vi "setMode.vi"(8 "error in (no error)":errorcluster, 10 "Mode":T1, 11 "Multimeter in":refnum<class "Multimeter.lvclass">) -> (0 "error out":errorcluster, 3 "Multimeter out":refnum<class "Multimeter.lvclass">)   [LabVIEW 2023, in "sweDmm.lvlib" / "Multimeter.lvclass"]
doc: "specify what the Dmm should measure."
uses:
  Multimeter.lvclass
  Data/DmmModes.ctl
  Multimeter.lvclass/Multimeter.ctl
  sweDmm.lvlib
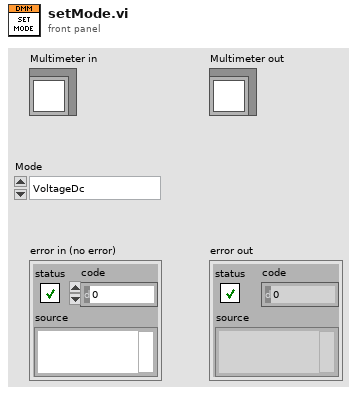
[diagram p1: front panel]
types:
  T1 = typedef "sweDmm.lvlib/DmmModes.ctl" = enum16{"VoltageDc", "VoltageAc", "CurrentDc", "CurrentAc", "Resistance2W"}
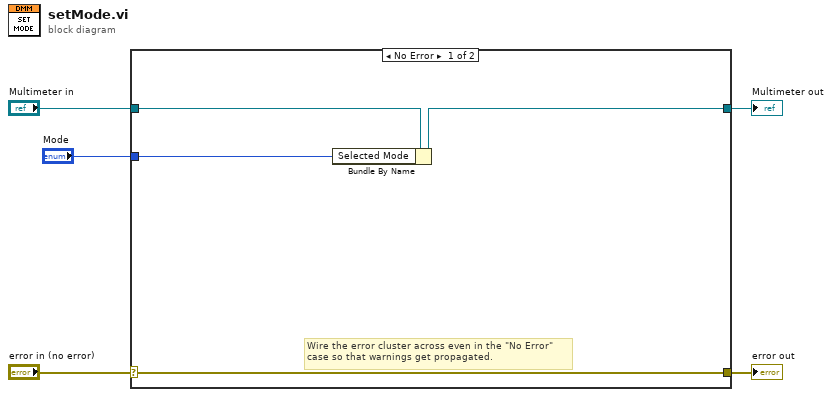
[diagram p0: block diagram]
diagram:
  n1 = case shown="No Error" "error in (no error)" {
    selector: "error in (no error)" -> [w8 w11]
    tunnel: [w8 w11] -> w4
    tunnel: [w7 w10] -> w2
    tunnel: "Multimeter in" -> [w9 w10]
    tunnel: "Mode" -> [w6 _]
    frame No Error {
      # "Wire the error cluster across even in the \"No Error\"\ncase so that warnings get propagated."
      n2 = Bundle By Name(cluster=w9, "Selected Mode"=w6) -> (w7:refnum<class "Multimeter.lvclass">)
    }
    frame Error {
    }
  }
  "error out" <- w4
  "Multimeter out" <- w2
